vi "add_amp_char_to_report.vi"(8 "error in (no error)":errorcluster, 11 "Boc12 in":refnum<class "Boc12.lvclass">) -> (0 "error out":errorcluster, 3 "Boc12 out":refnum<class "Boc12.lvclass">)   [LabVIEW 2017, in "Boc12.lvclass"]
uses:
  Boc12.lvclass
  home/andrew/projects/labview/boc/boc_setup/classes/report/Report.lvclass
  Report.lvclass/Report.ctl
  <vilib>/Utility/NIReport.llb/Append Text Table to Report (wrap).vi
  <vilib>/Utility/NIReport.llb/NI_report.lvclass
  Report.lvclass
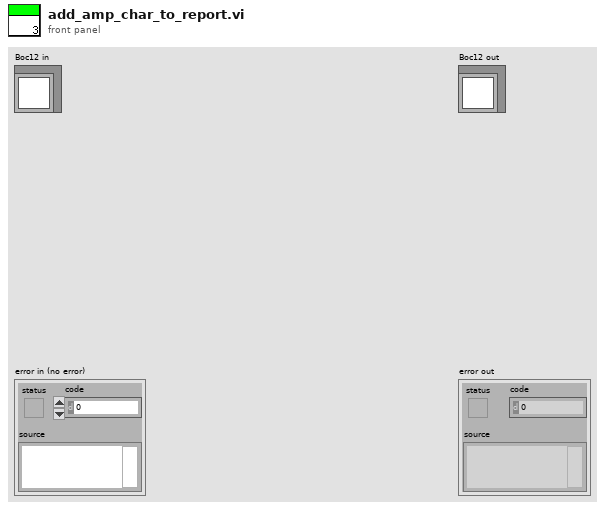
[diagram p1: front panel]
types:
  T1 = cluster{"position (excel)":cluster{"row":i32, "column":i32}, "name (excel)":string, "bookmark (word)":string}
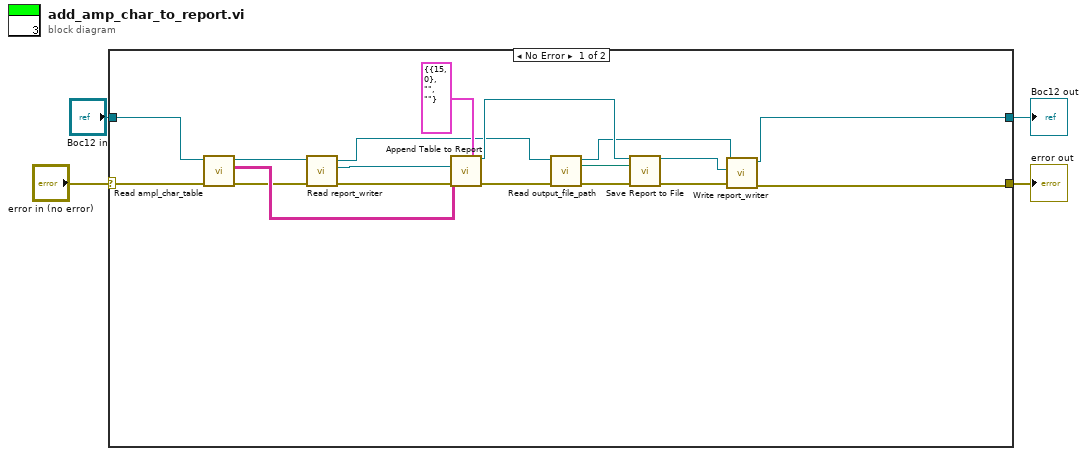
[diagram p0: block diagram]
diagram:
  n1 = case shown="No Error" "error in (no error)" {
    selector: "error in (no error)" -> [w16 w23]
    tunnel: "Boc12 in" -> [w17 w24]
    tunnel: [w6 w23] -> w2
    tunnel: [w5 w24] -> w1
    frame No Error {
      n2 = call-dynamic "Read ampl_char_table.vi"("error in (no error)"=w16, "Report in"=w17) -> ("error out"=w15:errorcluster, "ampl_char_table"=w18:string[][], "Report out"=w14:refnum<class "Boc12.lvclass">)  [unwired: 7 in]
      n3 = call "Read report_writer.vi"("error in (no error)"=w15, "Report in"=w14) -> ("error out"=w12:errorcluster, "NI_report.lvclass"=w13:refnum<class "NI_report.lvclass">, "Report out"=w11:refnum<class "Boc12.lvclass">)  [unwired: 7 in]
      n4 = call-poly <vilib>:"Append Table to Report.vi"("report in"=w13, "MS Office parameters"=T1 {"position (excel)"={"row"=15, "column"=0}, "name (excel)"="", "bookmark (word)"=""}, "text data"=w18, "error in (no error)"=w12) -> ("report out"=w21:refnum<class "NI_report.lvclass">, "error out"=w20:errorcluster)  [unwired: 8 in, 2 out]
      n5 = call "Read output_file_path.vi"("error in (no error)"=w20, "Report in"=w11) -> ("error out"=w19:errorcluster, "output_file_path"=w10:path, "Report out"=w8:refnum<class "Boc12.lvclass">)  [unwired: 7 in]
      n6 = call-dynamic "Save Report to File.vi"("report in"=w21, "report file path"=w10, "error in (no error)"=w19) -> ("report out"=w9:refnum<class "NI_report.lvclass">, "error out"=w7:errorcluster)  [unwired: 11 in]
      n7 = call "Write report_writer.vi"("error in (no error)"=w7, "NI_report.lvclass"=w9, "Report in"=w8) -> ("error out"=w6:errorcluster, "Report out"=w5:refnum<class "Boc12.lvclass">)  [unwired: 7 in]
    }
    frame Error {
    }
  }
  "error out" <- w2
  "Boc12 out" <- w1
